vi "Configure Hardware.vi"(8 "error in (no error)":errorcluster, 11 "Hardware Resources in":T1) -> (0 "error out":errorcluster, 3 "Hardware Resources out":T1)   [LabVIEW 2024, in "DAQ_msgHandler Acquisition.lvlib"]
doc: "Configure the hardware."
uses:
  DAQ_msgHandler Acquisition.lvlib
  Hardware Configuration.ctl
  Signal Type.ctl
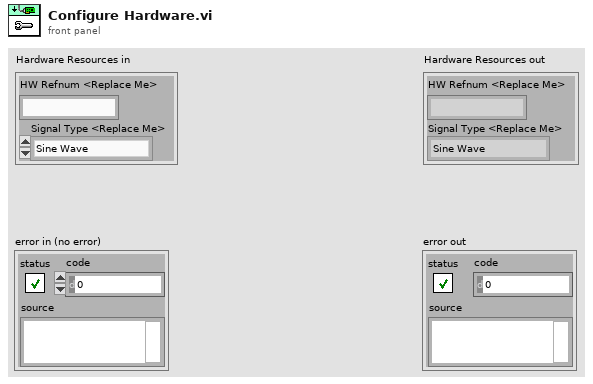
[diagram p1: front panel]
types:
  T1 = typedef "DAQ_msgHandler Acquisition.lvlib/Hardware Configuration.ctl" = cluster{"HW Refnum <Replace Me>":string, "Signal Type <Replace Me>":T2}
  T2 = typedef "DAQ_msgHandler Acquisition.lvlib/Signal Type.ctl" = enum16{"Sine Wave", "Square with Noise"}
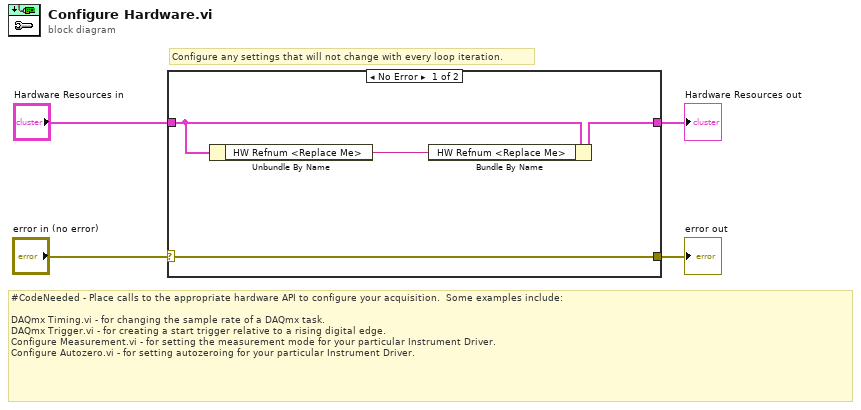
[diagram p0: block diagram]
diagram:
  # "Configure any settings that will not change with every loop iteration."
  # "#CodeNeeded - Place calls to the appropriate hardware API to configure your acquisition.  Some examples include:\n\nDAQmx Timing.vi - for changing the sample rate of a DAQmx task.\nDAQmx Trigger.vi - for creating a start trigger relative to a rising digital edge.\nConfigure Measurement.vi - for setting the measurement mode for your particular Instrument Driver.\nConfigure Autozero.vi - for setting autozeroing for your particular Instrument Driver."
  n1 = case shown="No Error" "error in (no error)" {
    selector: "error in (no error)" -> [w7 w9]
    tunnel: [w7 w9] -> w3
    tunnel: "Hardware Resources in" -> [w6 w10]
    tunnel: [w8 w10] -> w1
    frame No Error {
      n2 = Unbundle By Name(w6) -> ("HW Refnum <Replace Me>"=w5:string)
      n3 = Bundle By Name(cluster=w6, "HW Refnum <Replace Me>"=w5) -> (w8:T1)
    }
    frame Error {
    }
  }
  "Hardware Resources out" <- w1
  "error out" <- w3
